vi "acuqure multi subvi.vi"(7 "Array 6":string[](array[string])=["5ns", "10ns", "20ns", "50ns", "100ns", "200ns", "500ns", "1us", "2us", "5us", "10us", "20us", "50us", "100us", "200us", "500us", "1ms", "2ms", "5ms", "10ms", "20ms", "50ms", "100ms", "200ms", "500ms", "1s", "2s", "5s", "10s", "20s", "50s", "100s"], 9 "read buffer 2":string, 10 "read buffer":string) -> (1 "Waveform Graph":i8[][](graph), 2 "unsigned 16bit integer":u16, 3 "CH2 precision":string, 4 "CH1 precision":string, 5 "M":string)   [LabVIEW 2023, in "owon.lvlib"]
uses:
  owon.lvlib
panel:
  in  "Array 11":string[](array[string])=["2v", "5v", "10v", "20v", "50v", "100v", "200v", "500v", "1kv", "2kv", "5kv", "10kv", "0", "0", "0", "0", "0", "0", "0", "0"]
  in  "Array 10":string[](array[string])=["200mv", "500mv", "1v", "2v", "5v", "10v", "20v", "50v", "100v", "200v", "500v", "1kv", "0", "0", "0", "0", "0", "0", "0", "0"]
  in  "Array 9":string[](array[string])=["20mv", "50mv", "100mv", "200mv", "500mv", "1v", "2v", "5v", "10v", "20v", "50v", "100v", "0", "0", "0", "0", "0", "0", "0", "0"]
  in  "Array 8":string[](array[string])=["2mv", "5mv", "10mv", "20mv", "50mv", "100mv", "200mv", "500mv", "1v", "2v", "5v", "10v", "0", "0", "0", "0", "0", "0", "0", "0"]
  in  "Array 7":string[](array[string])=["2v", "5v", "10v", "20v", "50v", "100v", "200v", "500v", "1kv", "2kv", "5kv", "10kv", "0", "0", "0", "0", "0", "0", "0", "0"]
  in  "Array 5":string[](array[string])=["200mv", "500mv", "1v", "2v", "5v", "10v", "20v", "50v", "100v", "200v", "500v", "1kv", "0", "0", "0", "0", "0", "0", "0", "0"]
  in  "Array 4":string[](array[string])=["20mv", "50mv", "100mv", "200mv", "500mv", "1v", "2v", "5v", "10v", "20v", "50v", "100v", "0", "0", "0", "0", "0", "0", "0", "0"]
  in  "Array 2":string[](array[string])=["2mv", "5mv", "10mv", "20mv", "50mv", "100mv", "200mv", "500mv", "1v", "2v", "5v", "10v", "0", "0", "0", "0", "0", "0", "0", "0"]
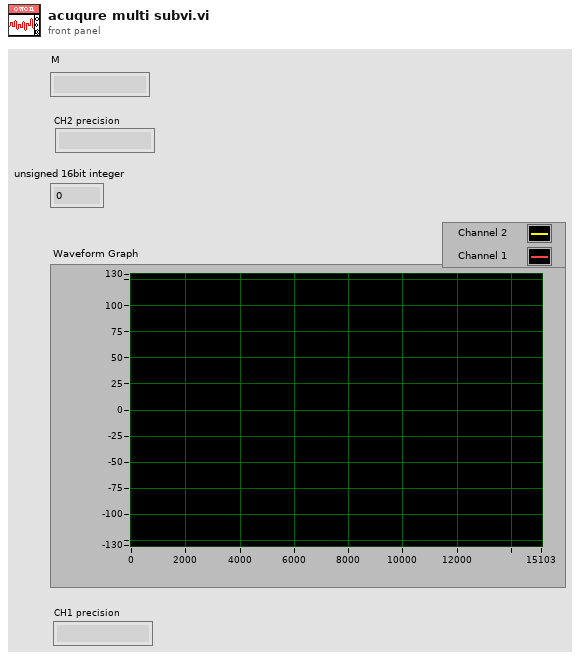
[diagram p1: front panel]
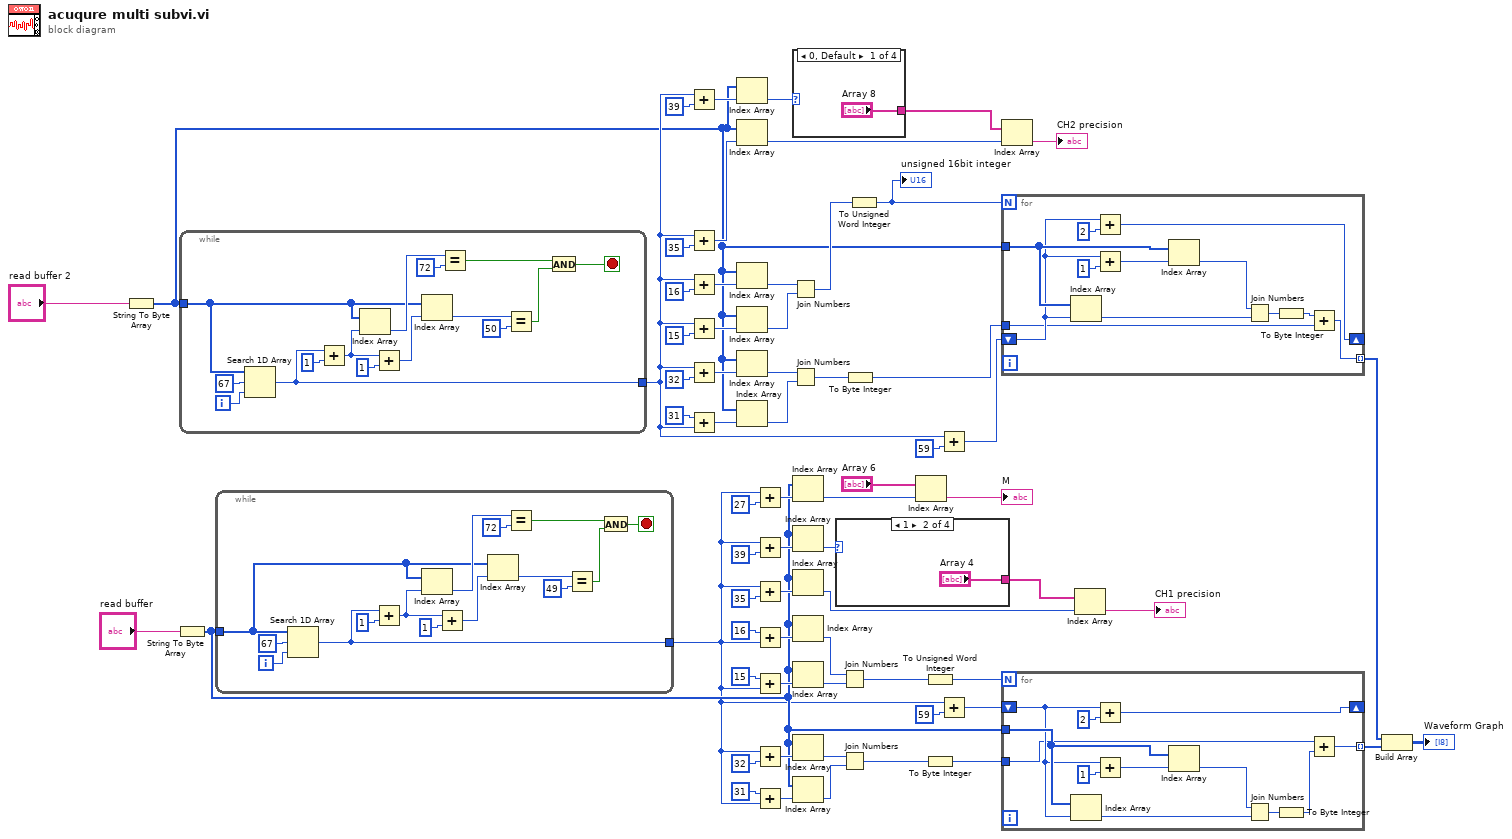
[diagram p0: block diagram]
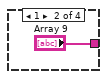
[diagram p2: hidden frame]
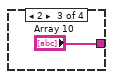
[diagram p3: hidden frame]
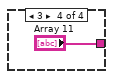
[diagram p4: hidden frame]
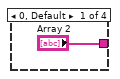
[diagram p5: hidden frame]
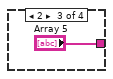
[diagram p6: hidden frame]
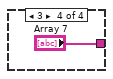
[diagram p7: hidden frame]
diagram:
  n1 = String To Byte Array(string="read buffer 2") -> (unsigned byte array=w2:u8[])
  n2 = String To Byte Array(string="read buffer") -> (unsigned byte array=w9:u8[])
  n3 = while {
    tunnel: [w77] -> w3
    tunnel: w2 -> [w70]
    i -> [w78]
    stop <- w72 stop-if-true
    n4 = Search 1D Array(1D array=w70, element=u8 67 ("元素"), start index (0)=w78) -> (index of element=w77:i32)
    n5 = Add(x=w77, y=1) -> (x+y=w71:i32)
    n6 = Index Array(array=w70, index=w71) -> (element=w75:u8)
    n7 = Add(x=w71, y=1) -> (x+y=w69:i32)
    n8 = Index Array(array=w70, index=w69) -> (element=w68:u8)
    n9 = Equal?(x=w75, y=u8 72 ("元素")) -> (x = y?=w73:bool)
    n10 = Equal?(x=w68, y=u8 50) -> (x = y?=w74:bool)
    n11 = And(x=w73, y=w74) -> (x .and. y?=w72:bool)
  }
  n12 = while {
    tunnel: [w91] -> w8
    tunnel: w9 -> [w84]
    i -> [w92]
    stop <- w86 stop-if-true
    n13 = Search 1D Array(1D array=w84, element=u8 67 ("元素"), start index (0)=w92) -> (index of element=w91:i32)
    n14 = Add(x=w91, y=1) -> (x+y=w89:i32)
    n15 = Index Array(array=w84, index=w89) -> (element=w94:u8)
    n16 = Add(x=w89, y=1) -> (x+y=w85:i32)
    n17 = Index Array(array=w84, index=w85) -> (element=w83:u8)
    n18 = Equal?(x=w94, y=u8 72 ("元素")) -> (x = y?=w87:bool)
    n19 = Equal?(x=w83, y=u8 49) -> (x = y?=w88:bool)
    n20 = And(x=w87, y=w88) -> (x .and. y?=w86:bool)
  }
  n21 = Add(x=w3, y=39) -> (x+y=w6:i32)
  n22 = Add(x=w3, y=35) -> (x+y=w23:i32)
  n23 = Add(x=w3, y=16 ("x")) -> (x+y=w66:i32)
  n24 = Add(x=w3, y=15) -> (x+y=w59:i32)
  n25 = Add(x=w3, y=32) -> (x+y=w17:i32)
  n26 = Add(x=31, y=w3) -> (x+y=w15:i32)
  n27 = Index Array(array=w2, index=w6) -> (element=w4:u8)
  n28 = Index Array(array=w2, index=w23) -> (element=w24:u8)
  n29 = Index Array(array=w2, index=w66) -> (element=w62:u8)
  n30 = Index Array(array=w2, index=w59) -> (element=w61:u8)
  n31 = Index Array(array=w2, index=w17) -> (element=w20:u8)
  n32 = Index Array(array=w2, index=w15) -> (element=w19:u8)
  n33 = Add(x=w8, y=27) -> (x+y=w41:i32)
  n34 = Add(x=w8, y=39) -> (x+y=w12:i32)
  n35 = Add(x=w8, y=35) -> (x+y=w38:i32)
  n36 = Add(x=16, y=w8) -> (x+y=w51:i32)
  n37 = Add(x=15, y=w8) -> (x+y=w52:i32)
  n38 = Add(x=w8, y=32) -> (x+y=w32:i32)
  n39 = Add(x=31, y=w8) -> (x+y=w30:i32)
  n40 = Join Numbers(hi=w62, lo=w61) -> ((hi.lo)=w63:u16)
  n41 = Join Numbers(hi=w20, lo=w19) -> ((hi.lo)=w21:u16)
  n42 = case shown="0, Default" w4 {
    tunnel: ["Array 8" "Array 9" "Array 10" "Array 11"] -> w1
    frame 0, Default {
    }
    frame 1 {
    }
    frame 2 {
    }
    frame 3 {
    }
  }
  n43 = Index Array(array=w9, index=w41) -> (element=w42:u8)
  n44 = Index Array(array=w9, index=w12) -> (element=w10:u8)
  n45 = Index Array(array=w9, index=w38) -> (element=w39:u8)
  n46 = Index Array(array=w9, index=w51) -> (element=w55:u8)
  n47 = Index Array(array=w9, index=w52) -> (element=w56:u8)
  n48 = Index Array(array=w9, index=w32) -> (element=w35:u8)
  n49 = Index Array(array=w9, index=w30) -> (element=w34:u8)
  n50 = case shown="1" w10 {
    tunnel: ["Array 2" "Array 4" "Array 5" "Array 7"] -> w7
    frame 0, Default {
    }
    frame 1 {
    }
    frame 2 {
    }
    frame 3 {
    }
  }
  n51 = Join Numbers(hi=w55, lo=w56) -> ((hi.lo)=w57:u16)
  n52 = Join Numbers(hi=w35, lo=w34) -> ((hi.lo)=w36:u16)
  n53 = To Byte Integer(number=w21) -> (8bit integer=w25:i8)
  n54 = To Unsigned Word Integer(number=w63) -> (unsigned 16bit integer=w64:u16)
  "unsigned 16bit integer" <- w64
  n55 = Index Array(array="Array 6", index=w42) -> (element=→"M":string)
  n56 = To Unsigned Word Integer(number=w57) -> (unsigned 16bit integer=w58:u16)
  n57 = To Byte Integer(number=w36) -> (8bit integer=w43:i8)
  n58 = Add(x=w3, y=59) -> (x+y=w26:i32)
  n59 = Add(x=w8, y=59) -> (x+y=w44:i32)
  n60 = Index Array(array=w1, index=w24) -> (element=→"CH2 precision":string)
  n61 = for {
    N: w64 -> [_]
    tunnel: w2 -> [w116]
    shift-right: [w113] -> _
    shift-left: w26 -> [w112]
    tunnel: [w108] -> w13 mode=indexing
    tunnel: w25 -> [w105]
    n62 = Index Array(array=w116, index=w112) -> (element=w107:u8)
    n63 = Add(x=w112, y=2) -> (x+y=w113:i32)
    n64 = Add(x=w112, y=1) -> (x+y=w115:i32)
    n65 = Index Array(array=w116, index=w115) -> (element=w106:u8)
    n66 = Join Numbers(hi=w106, lo=w107) -> ((hi.lo)=w110:u16)
    n67 = To Byte Integer(number=w110) -> (8bit integer=w109:i8)
    n68 = Add(x=w109, y=w105) -> (x+y=w108:i8)
  }
  n69 = for {
    N: w58 -> [_]
    tunnel: w9 -> [w128]
    shift-right: [w125] -> _
    shift-left: w44 -> [w124]
    tunnel: [w120] -> w49 mode=indexing
    tunnel: w43 -> [w117]
    n70 = Index Array(array=w128, index=w124) -> (element=w118:u8)
    n71 = Add(x=w124, y=2) -> (x+y=w125:i32)
    n72 = Add(x=w124, y=1) -> (x+y=w127:i32)
    n73 = Index Array(array=w128, index=w127) -> (element=w119:u8)
    n74 = Join Numbers(hi=w119, lo=w118) -> ((hi.lo)=w122:u16)
    n75 = To Byte Integer(number=w122) -> (8bit integer=w121:i8)
    n76 = Add(x=w117, y=w121) -> (x+y=w120:i8)
  }
  n77 = Index Array(array=w7, index=w39) -> (element=→"CH1 precision":string)
  n78 = Build Array(w13, w49) -> (→"Waveform Graph":i8[][])
